vi "Threshold FPGA.vi"() -> ()   [LabVIEW 2010]
uses:
  <vilib>/eio/EIONode/EIONode.xnode
panel:
  in  "Stop FPGA":bool
  out "Threshold Exceeded":bool
  in  "Threshold (binary)":i16
  out "AI0 (binary)":i16
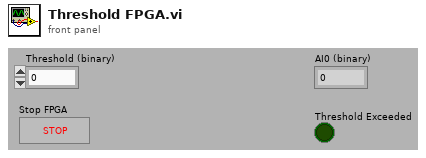
[diagram p1: front panel]
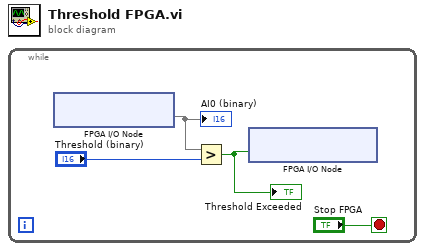
[diagram p0: block diagram]
diagram:
  n1 = while {
    stop <- "Stop FPGA" stop-if-true
    n2 = xnode "FPGA I/O Node"() -> ("Connector0/AI0"=w4)  [unwired: 1 in, 1 out]
    "AI0 (binary)" <- w4
    n3 = Greater?(x=w4, y="Threshold (binary)") -> (0:w3:bool)
    "Threshold Exceeded" <- w3
    n4 = xnode "FPGA I/O Node"("Connector0/DIO0"=w3) -> ()  [unwired: 1 in, 1 out]
  }
